vi "terminate.vi"(8 "error in (no error)":errorcluster, 11 "GenericPlugin in":refnum<class "FPGAWrapperRK110909Throughput.lvclass">) -> (0 "error out":errorcluster, 3 "GenericPlugin out":refnum<class "FPGAWrapperRK110909Throughput.lvclass">)   [LabVIEW 2010, in "FPGAWrapperRK110909Throughput.lvclass"]
doc: "The dynamic dispatch version of this VI terminates the plug-in object by releasing all of its resources."
uses:
  FPGAWrapperRK110909Throughput.lvclass
  FPGA_reference.ctl
  <vilib>/rvi/interface/nirviReadWriteControl/nirviReadWriteControl.xnode
  <vilib>/rvi/interface/common/niFpgaNodeNameForErrorReporting.ctl
  <vilib>/rvi/errors/niLvFpgaWhatHappensToTopLevelVI.ctl
  <vilib>/rvi/interface/nirviCloseFPGA/nirviCloseFPGA.xnode
  GenericFPGAWrapper/GenericFPGAWrapper/GenericFPGAWrapper.lvclass
  <vilib>/Utility/error.llb/Error Cluster From Error Code.vi
  <vilib>/rvi/errors/niLvFpgaAdjustHostInterfaceError.vi
  <vilib>/FPGAPlugInAG/Dynamic/niLvFpga_Close_Dynamic.vi
  NiFpgaLv.dll
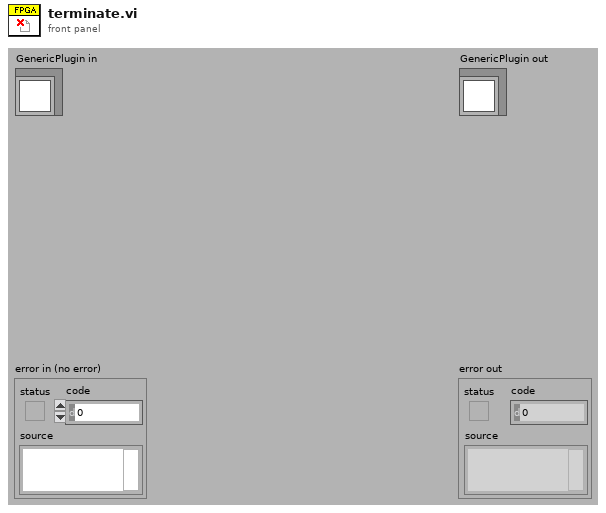
[diagram p1: front panel]
types:
  T1 = typedef "FPGAWrapperRK110909Throughput.lvclass/FPGA_reference.ctl" = refnum<k20>
  T2 = typedef "niFpgaNodeNameForErrorReporting.ctl" = enum16{"Open FPGA VI Reference", "Read/Write Control", "Invoke Method: Abort", "Invoke Method: Acknowledge IRQ", "Invoke Method: Download", "Invoke Method: FIFO.Configure", "Invoke Method: FIFO.Read", "Invoke Method: FIFO.Start", "Invoke Method: FIFO.Stop", "Invoke Method: FIFO.Write", "Invoke Method: Reset", "Invoke Method: Run", "Invoke Method: Wait on IRQ", "Close FPGA VI Reference"}
  T3 = typedef "niLvFpgaWhatHappensToTopLevelVI.ctl" = enum16{"top level VI scripted behind XNode", "top level VI inlined behind XNode"}
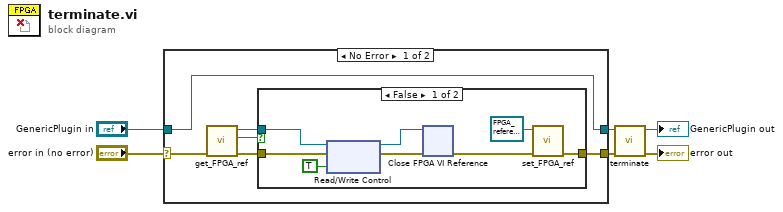
[diagram p0: block diagram]
diagram:
  n1 = case shown="No Error" "error in (no error)" {
    selector: "error in (no error)" -> [w12 w68]
    tunnel: "GenericPlugin in" -> [w7 w67]
    tunnel: [w8 w68] -> w2
    tunnel: [w7 w67] -> w1
    frame No Error {
      n2 = call "get_FPGA_ref.vi"("error in"=w12) -> ("error out"=w11:errorcluster, "Is empty?"=w10:bool, "FPGA Reference"=w9:T1)  [unwired: 8 in]
      n3 = case shown="False" w10 {
        tunnel: w11 -> [w17 w66]
        tunnel: w9 -> [w15 _]
        tunnel: [w20 w66] -> w8
        frame False {
          n4 = xnode "Read/Write Control"("FPGA VI Reference In"=w15, "error in"=w17, "Quit"=TRUE) -> ("FPGA VI Reference Out"=w14:T1, "error out"=w16:errorcluster)
          n5 = xnode "Close FPGA VI Reference"("FPGA VI Reference In"=w14, "error in"=w16) -> ("error out"=w19:errorcluster)
          n6 = call "set_FPGA_ref.vi"("error in"=w19, "FPGA Reference"=T1 refnum) -> ("error out"=w20:errorcluster)  [unwired: 9 in]
        }
        frame True {
        }
      }
    }
    frame Error {
    }
  }
  n7 = call-parent "terminate.vi"("error in (no error)"=w2, "GenericPlugin in"=w1) -> ("error out"=→"error out":errorcluster, "GenericPlugin out"=→"GenericPlugin out":refnum<class "FPGAWrapperRK110909Throughput.lvclass">)  [unwired: 8 in]
